vi "ScopeVoltage(SubVI).vi"(8 "error in (no error)":errorcluster, 11 "VISA Refnum in":refnum<visa-resource-name>) -> (0 "error out":errorcluster, 1 "Units":string, 2 "Measurement":dbl, 3 "VISA Refnum out":refnum<visa-resource-name>)   [LabVIEW 2013]
uses:
  <instrlib>/Tektronix TDS 200 1000 2000 Series/Tektronix TDS 200 1000 2000 Series.lvlib
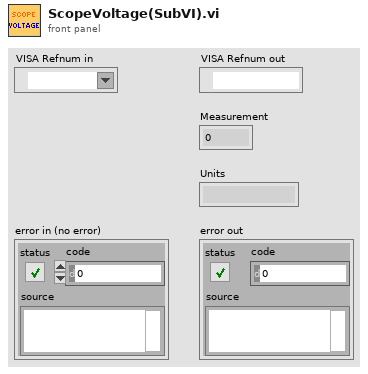
[diagram p1: front panel]
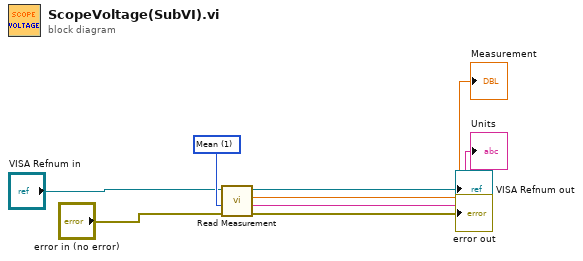
[diagram p0: block diagram]
diagram:
  w7 = u16 1 items=["Frequency", "Mean", "Period", "Pulse Duty", "Peak to Peak", "Complete RMS", "Minimum", "Maximum", "Rise Time", "Fall Time", "Positive Width", "Negative Width"] ("Measurement Type (0: Frequency)")
  n1 = call <instrlib>:"Read Measurement.vi"("error in (no error)"="error in (no error)", "Measurement Type (0: Frequency)"=w7, "VISA resource name"="VISA Refnum in") -> ("error out"=→"error out":errorcluster, "Units"=→"Units":string, "Measurement"=→"Measurement":dbl, "VISA resource name out"=→"VISA Refnum out":refnum<visa-resource-name>)  [unwired: 5 in]
